vi "Arduino_GetBoardListing.vi"() -> (2 "All Names":string[](array[string]))   [LabVIEW 2020]
panel:
  out "text":string
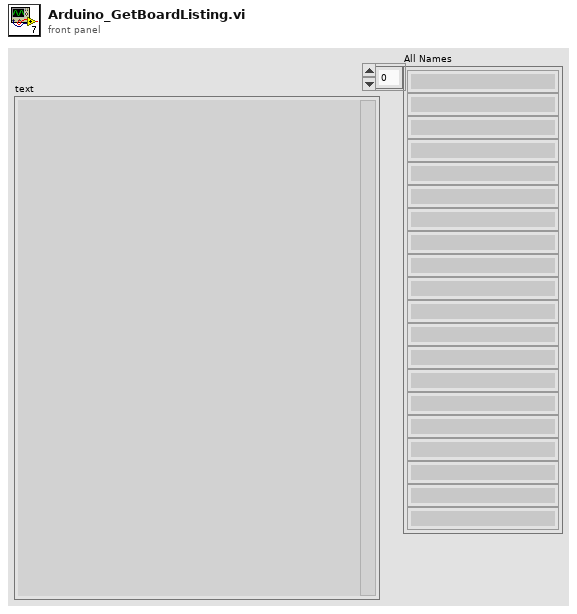
[diagram p1: front panel]
types:
  T1 = cluster{"packages":cluster{"name":string, "maintainer":string, "websiteURL":string, "platforms":cluster{"name":string, "architecture":string, "version":string, "category":string, "url":string, "archiveFileName":string, "checksum":string, "size":string, "boards":cluster{"name":string}[], "toolsDependencies":cluster{"packager":string, "name":string, "version":string}[]}[]}[]}
  T2 = cluster{"name":string, "maintainer":string, "websiteURL":string, "platforms":cluster{"name":string, "architecture":string, "version":string, "category":string, "url":string, "archiveFileName":string, "checksum":string, "size":string, "boards":cluster{"name":string}[], "toolsDependencies":cluster{"packager":string, "name":string, "version":string}[]}[]}[]
  T3 = cluster{"name":string, "architecture":string, "version":string, "category":string, "url":string, "archiveFileName":string, "checksum":string, "size":string, "boards":cluster{"name":string}[], "toolsDependencies":cluster{"packager":string, "name":string, "version":string}[]}[]
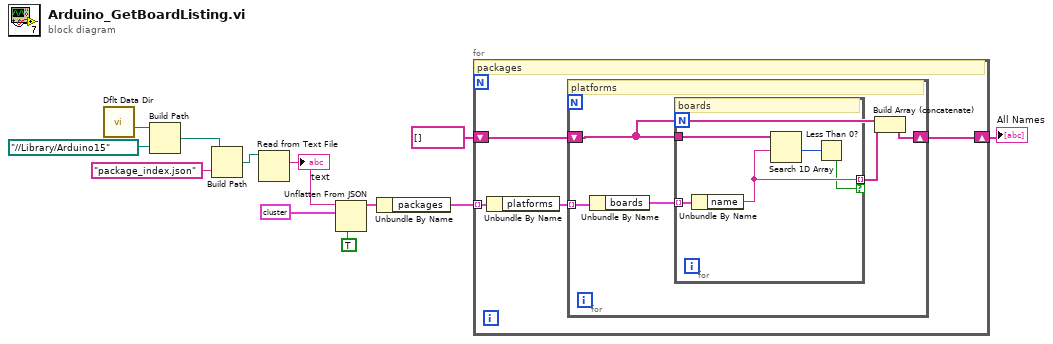
[diagram p0: block diagram]
diagram:
  n1 = call <vilib>:"Dflt Data Dir.vi"() -> ("App:Default Data Directory"=w12:path)
  n2 = Build Path(base path=w12, name or relative path=path "../../Library/Arduino15") -> (appended path=w4:path)
  n3 = Build Path(base path=w4, name or relative path="package_index.json") -> (appended path=w10:path)
  n4 = Read from Text File(file (use dialog)=w10) -> (text=w9:string)  [unwired: 3 in, 3 out]
  "text" <- w9
  n5 = Unflatten From JSON(JSON string=w9, type and defaults=T1 {"packages"=[{"name"="", "maintainer"="", "websiteURL"="", "platforms"=[{"name"=" ", "architecture"="", "version"="", "category"="", "url"="", "archiveFileName"="", "checksum"="", "size"="", "boards"=[{"name"=" "}], "toolsDependencies"=[{"packager"=" ", "name"="", "version"=""}]}]}]}, default null elements? (F)=TRUE) -> (value=w6:T1)  [unwired: 4 in, 1 out]
  n6 = Unbundle By Name(w6) -> ("packages"=w5:T2)
  n7 = for {
    tunnel: w5 -> [w15] mode=indexing
    shift-right: [w14] -> w3
    shift-left: string[] [] -> [w13]
    # "packages"
    n8 = Unbundle By Name(w15) -> ("platforms"=w16:T3)
    n9 = for {
      tunnel: w16 -> [w20] mode=indexing
      shift-right: [w17] -> w14
      shift-left: w13 -> [w19]
      # "platforms"
      n10 = Unbundle By Name(w20) -> ("boards"=w21:cluster{"name":string}[])
      n11 = for {
        tunnel: w21 -> [w26] mode=indexing
        tunnel: [w24] -> w18 mode=indexing if=w22
        tunnel: w19 -> [w25]
        # "boards"
        n12 = Unbundle By Name(w26) -> ("name"=w24:string)
        n13 = Search 1D Array(1D array=w25, element=w24) -> (index of element=w23:i32)  [unwired: 1 in]
        n14 = Less Than 0?(x=w23) -> (x < 0?=w22:bool)
      }
      n15 = Build Array (concatenate)(w19, w18) -> (w17:string[])
    }
  }
  "All Names" <- w3
